vi "ag33xxx - Select User Def Wfm.vi"(8 "error in (no error)":errorcluster, 9 "User Def. Wfm Name":string, 11 "VISA session":refnum<visa-resource-name>) -> (0 "error out":errorcluster, 3 "dup VISA session":refnum<visa-resource-name>)   [LabVIEW 2012]
doc: "Selects one of four user-defined waveforms. The Waveform name is required."
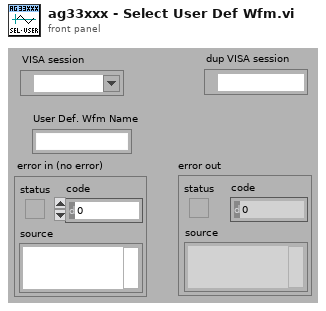
[diagram p1: front panel]
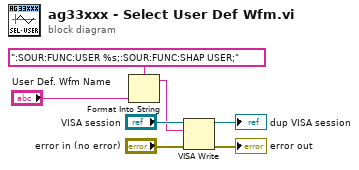
[diagram p0: block diagram]
diagram:
  n1 = Format Into String(format string=":SOUR:FUNC:USER %s;:SOUR:FUNC:SHAP USER;", "User Def. Wfm Name") -> (resulting string=w1:string)  [unwired: 2 in, 1 out]
  n2 = VISA Write(VISA resource name="VISA session", write buffer=w1, error in (no error)="error in (no error)") -> (VISA resource name out=→"dup VISA session":refnum<visa-resource-name>, error out=→"error out":errorcluster)  [unwired: 1 out]
